vi "INTELLIFAUCET Get Micro Amp Value.vi"(7 "uA Set":i32, 8 "error in (no error)":errorcluster, 9 "Temp/GPM Target":dbl=58.0 format="%#_13g", 10 "Use General Conversion":bool, 11 "TEMP,FLOW in":T1=enum."FLOW") -> (0 "error out":errorcluster, 2 "TEMP,FLOW out":T1, 3 "uA Output":i32)   [LabVIEW 2023]
uses:
  Type Definitions/INTELLIFAUCT Temp Flow.ctl
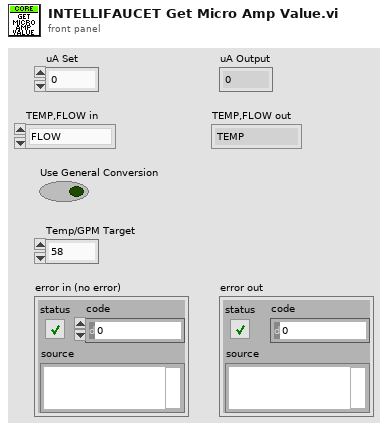
[diagram p1: front panel]
types:
  T1 = typedef "INTELLIFAUCT Temp Flow.ctl" = enum8{"TEMP", "FLOW", "Prop Valve"}
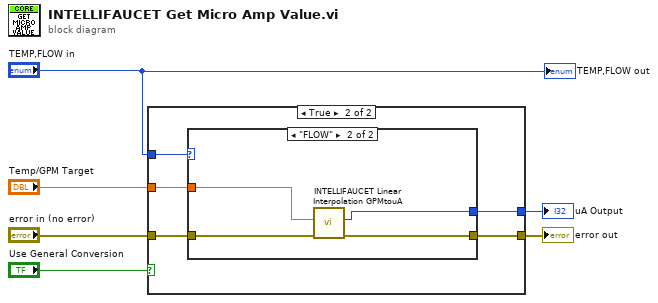
[diagram p0: block diagram]
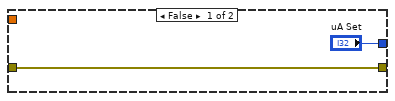
[diagram p2: hidden frame]
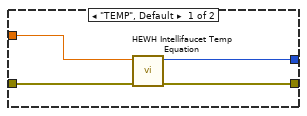
[diagram p3: hidden frame]
diagram:
  n1 = case shown="True" "Use General Conversion" {
    tunnel: "Temp/GPM Target" -> [_ w13]
    tunnel: ["uA Set" w12] -> w3
    tunnel: "error in (no error)" -> [w7 w11]
    tunnel: [w7 w10] -> w5
    tunnel: "TEMP,FLOW in" -> [_ w9]
    frame False {
    }
    frame True {
      n2 = case shown="\"FLOW\"" w9 {
        tunnel: w11 -> [w15 w21]
        tunnel: w13 -> [w17 w20]
        tunnel: [w14 w19] -> w10
        tunnel: [w16 w18] -> w12
        frame "TEMP", Default {
          n3 = call "HEWH Intellifaucet Temp Equation.vi"("Error In"=w15, "Temp/GPM Target"=w17) -> ("Error Out"=w14:errorcluster, "Temp uA"=w16:i32)  [unwired: 7 in, 1 out]
        }
        frame "FLOW" {
          n4 = call "INTELLIFAUCET Linear Interpolation GPMtouA.vi"("Error In"=w21, "Target"=w20) -> ("Error Out"=w19:errorcluster, "uA Output"=w18:i32)  [unwired: 8 in]
        }
      }
    }
  }
  "error out" <- w5
  "uA Output" <- w3
  "TEMP,FLOW out" <- "TEMP,FLOW in"
